vi "Stop Core.vi"(10 "final error code":i32, 11 "SPIController in":refnum<class "SPIController.lvclass">) -> (3 "SPIController out":refnum<class "SPIController.lvclass">)   [LabVIEW 2023, in "SPIController.lvlib" / "SPIController.lvclass"]
doc: "(<B>Filename</B>: Actor Framework.lvlib:Actor.lvclass:Stop Core.vi)\n\nDefines what the actor does before it stops. Use the <B>final error code</B> input to determine whether the actor shut down in response to an error.\n\nBy default, this method passes the Stop message along to all auto-stop nested actors. A descendant class may override this method to define additional behavior, such as shutting down any processes the actor initiated in its override of the Actor Core method."
uses:
  SPIController.lvclass
  SPIController.lvclass/SPIController.ctl
  <vilib>/ActorFramework/Actor/Actor.lvclass
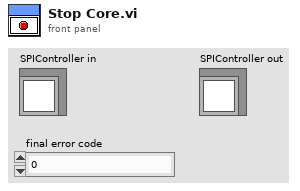
[diagram p1: front panel]
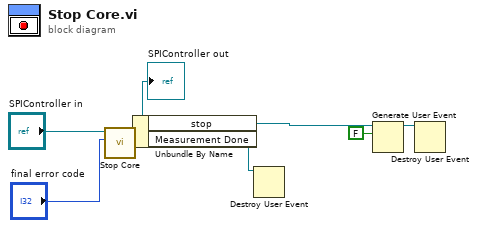
[diagram p0: block diagram]
diagram:
  n1 = call-parent "Stop Core.vi"("final error code"="final error code", "Actor in"="SPIController in") -> ("Actor out"=w5:refnum<class "SPIController.lvclass">)  [unwired: 9 in]
  "SPIController out" <- w5
  n2 = Unbundle By Name(w5) -> ("stop"=w4:refnum<user-event>, "Measurement Done"=w2:refnum<user-event>)
  n3 = Destroy User Event(user event=w2) -> ()  [unwired: 1 in, 1 out]
  n4 = Generate User Event(user event=w4, event data cluster=FALSE ("event data")) -> (user event out=w3:refnum<user-event>)  [unwired: 2 in, 1 out]
  n5 = Destroy User Event(user event=w3) -> ()  [unwired: 1 in, 1 out]
